vi "PID Output Rate Limiter.vi"   [LabVIEW 2020, in "NI_PID_pid.lvlib"]
doc: "Limits the rate of change of the controller output. Place this VI immediately after the PID VI in your control application. Use the DBL instance of this VI to implement a single control loop. Use the DBL Array instance to implement parallel multi-loop control."
uses:
  NI_PID_pid.lvlib
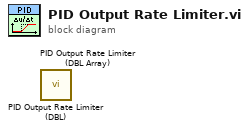
[diagram p0: block diagram]
diagram:
  n1 = call "PID Output Rate Limiter (DBL).vi"() -> ()  [unwired: 8 in, 2 out]
  n2 = call "PID Output Rate Limiter (DBL Array).vi"() -> ()  [unwired: 8 in, 2 out]
